vi "SeqMgr.Math Statement Execute.vi"(10 "Arguements":string[](array[string])) -> (2 "Vars Out":string[][](array[string]))   [LabVIEW 2024, in "EQMF.lvlib" / "SeqMgr.lvlib"]
uses:
  SeqMgr.lvlib
  <vilib>/Utility/error.llb/Trim Whitespace One-Sided.vi
panel:
  # "Math(Result,Value1,Oper,Value2)\nName = Value Oper Value"
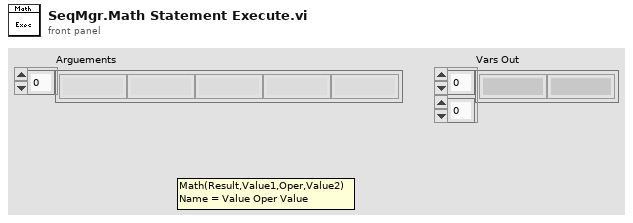
[diagram p1: front panel]
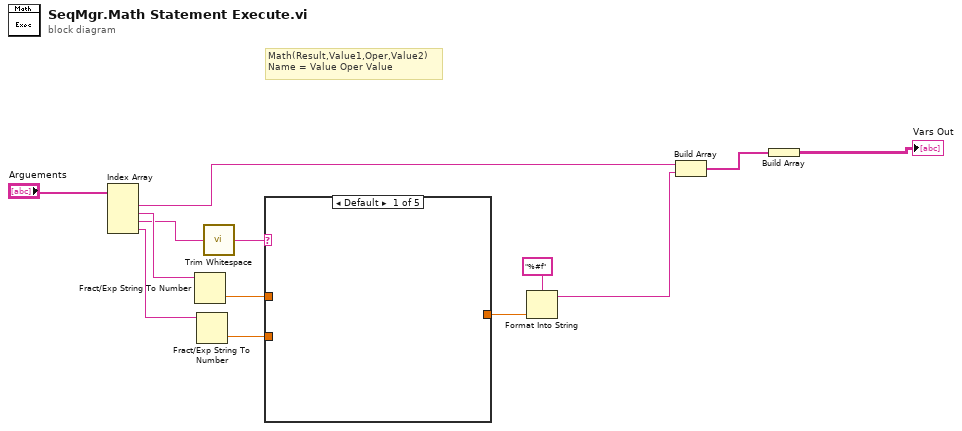
[diagram p0: block diagram]
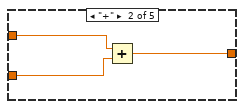
[diagram p2: hidden frame]
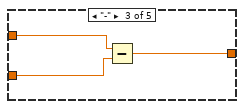
[diagram p3: hidden frame]
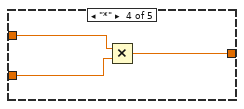
[diagram p4: hidden frame]
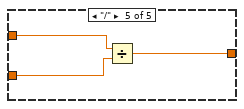
[diagram p5: hidden frame]
diagram:
  # "Math(Result,Value1,Oper,Value2)\nName = Value Oper Value"
  n1 = Index Array(array="Arguements") -> (element #1=w10:string, element #2=w9:string, element #3=w5:string, element #4=w8:string)  [unwired: 4 in]
  n2 = Fract/Exp String To Number(string=w9) -> (number=w7:dbl)  [unwired: 3 in, 1 out]
  n3 = Fract/Exp String To Number(string=w8) -> (number=w6:dbl)  [unwired: 3 in, 1 out]
  n4 = call <vilib>:"Trim Whitespace.vi"("string"=w5) -> ("trimmed string"=w4:string)  [unwired: 1 in]
  n5 = case shown="Default" w4 {
    tunnel: w7 -> [_ w16 w19 w22 w25]
    tunnel: w6 -> [_ w15 w18 w21 w24]
    tunnel: [_ w14 w17 w20 w23] -> w3
    frame Default {
    }
    frame "+" {
      n6 = Add(x=w16, y=w15) -> (x+y=w14:dbl)
    }
    frame "-" {
      n7 = Subtract(x=w19, y=w18) -> (x-y=w17:dbl)
    }
    frame "*" {
      n8 = Multiply(x=w22, y=w21) -> (x*y=w20:dbl)
    }
    frame "/" {
      n9 = Divide(x=w25, y=w24) -> (x/y=w23:dbl)
    }
  }
  n10 = Format Into String(format string="%#f", w3) -> (resulting string=w1:string)  [unwired: 2 in, 1 out]
  n11 = Build Array(w10, w1) -> (w12:string[])
  n12 = Build Array(w12) -> (→"Vars Out":string[][])
